vi "Start BuildWorker.vi"(8 "error in (no error)":errorcluster, 9 "Show":bool=TRUE, 10 "Port":i32=4545, 11 "BuildWorker Basics in":refnum<class "BuildWorker Basics.lvclass">) -> (0 "error out":errorcluster, 3 "BuildWorker Basics out":refnum<class "BuildWorker Basics.lvclass">)   [LabVIEW 2017, in "BuildWorker Interface.lvlib" / "BuildWorker Basics.lvclass"]
uses:
  BuildWorker Basics.lvclass
  BuildWorker Basics.lvclass/BuildWorker Basics.ctl
  <vilib>/ActorFramework/Message Enqueuer/Message Enqueuer.lvclass
panel:
  out "App.ContextName":string
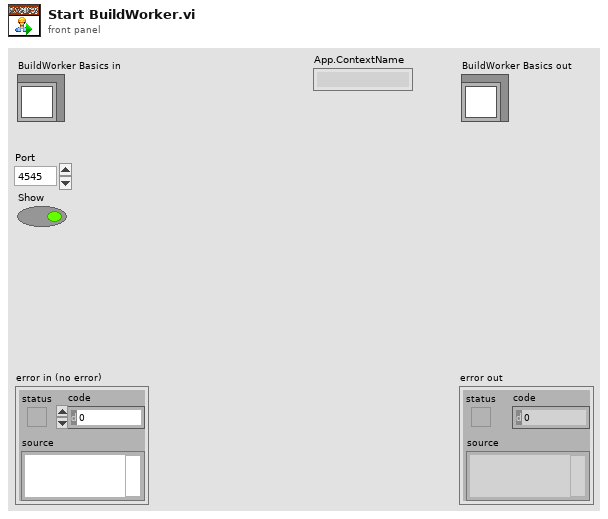
[diagram p1: front panel]
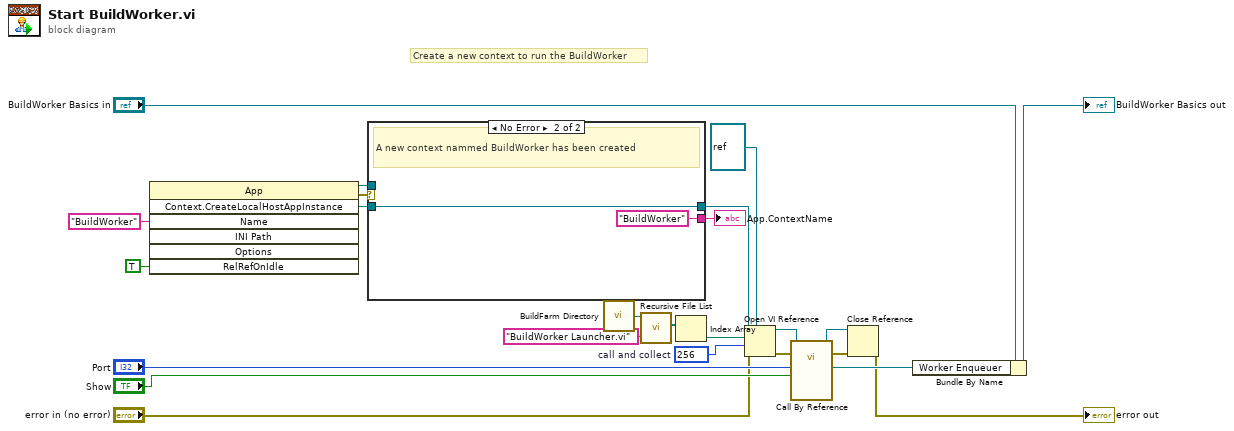
[diagram p0: block diagram]
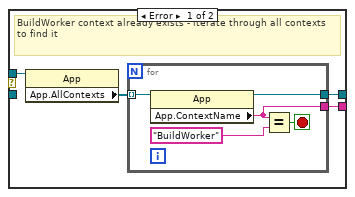
[diagram p2: hidden frame]
diagram:
  w22 = 256  # call and collect
  # "Create a new context to run the BuildWorker"
  n1 = invoke class="App" method="Context.CreateLocalHostAppInstance"("Name"="BuildWorker" ("Application Instance Name"), "RelRefOnIdle"=TRUE ("Release Ref on Idle (T)")) -> (reference out=w7:refnum<vi>, error out=w10:errorcluster, "Create Context"=w9:refnum<vi>)  [unwired: 5 in, 4 out]
  n2 = case shown="No Error" w10 {
    tunnel: w9 -> [_ w35]
    tunnel: [w26 w35] -> w8
    tunnel: w7 -> [w28 _]
    tunnel: [w25 "BuildWorker" ("App.ContextName")] -> w1
    frame Error {
      # "BuildWorker context already exists - iterate through all contexts to find it"
      n3 = property class="App"(reference=w28) -> ("App.AllContexts"=w27:refnum<vi>[])  [unwired: 1 in, 2 out]
      n4 = for {
        tunnel: w27 -> [w33] mode=indexing
        tunnel: [w30] -> w26
        tunnel: [w29] -> w25
        stop <- w31 stop-if-true
        n5 = property class="App"(reference=w33) -> (reference out=w30:refnum<vi>, "App.ContextName"=w29:string)  [unwired: 1 in, 1 out]
        n6 = Equal?(x=w29, y="BuildWorker" ("Application Instance Name")) -> (x = y?=w31:bool)
      }
    }
    frame No Error {
      # "A new context nammed BuildWorker has been created"
    }
  }
  "App.ContextName" <- w1
  n7 = call "BuildFarm Directory.vi"() -> ("BuildFarm Directory"=w16:path)
  n8 = call <vilib>:"Recursive File List.vi"("pattern"="BuildWorker Launcher.vi" ("VI Path"), "Folder Path"=w16) -> ("All Files in Dir"=w18:path[])  [unwired: 5 in, 4 out]
  n9 = Index Array(array=w18) -> (element=w17:path)  [unwired: 1 in]
  n10 = Open VI Reference(type specifier VI Refnum (for type only)=refnum<vi> refnum, application reference (local)=w8, vi path=w17, options=w22, error in (no error)="error in (no error)") -> (vi reference=w21:refnum<vi>, error out=w14:errorcluster)  [unwired: 1 in]
  n11 = call-by-ref "?"(reference=w21, error in=w14, "Show"="Show", "Port"="Port") -> (reference out=w20:refnum<vi>, error out=w13:errorcluster, "Worker Enqueuer"=w4:refnum<class "Message Enqueuer.lvclass">)  [unwired: 9 in]
  n12 = Close Reference(reference=w20, error in (no error)=w13) -> (error out=→"error out":errorcluster)
  n13 = Bundle By Name(cluster="BuildWorker Basics in", "Worker Enqueuer"=w4) -> (→"BuildWorker Basics out":refnum<class "BuildWorker Basics.lvclass">)
